vi "Read AI Channels.vi"(8 "error in (no error)":errorcluster, 11 "Task in":refnum<k21>) -> (0 "error out":errorcluster, 2 "1-Sample Average Waveforms":waveform(dbl)[](array[waveform]), 3 "Task out":refnum<k21>)   [LabVIEW 2021, in "Load Frame.lvlib"]
uses:
  Load Frame.lvlib
  <vilib>/DAQmx/miscellaneous.llb/DAQmx Fill In Error Info.vi
  <vilib>/DAQmx/read.llb/DAQmx Read (Analog 1D Wfm NChan NSamp).vi
  Acquisition/Acquisition.lvlib
  <vilib>/DAQmx/read.llb/DAQmx Read (Analog 1D Wfm NChan 1Samp).vi
panel:
  out "Unscaled Data":waveform(dbl)[](graph)
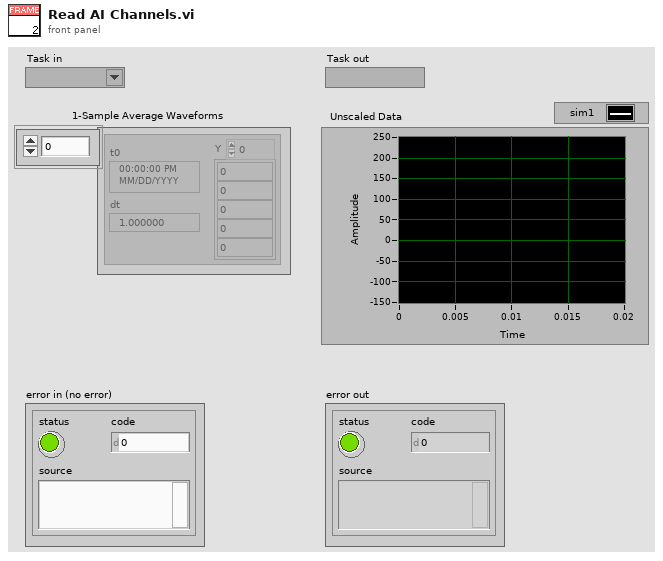
[diagram p1: front panel]
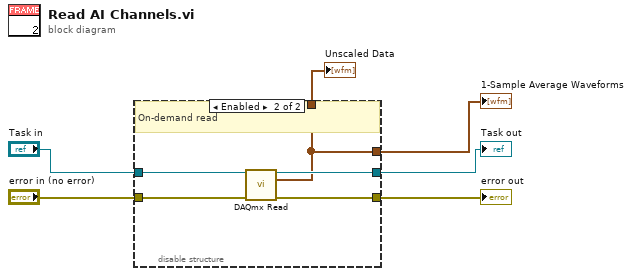
[diagram p0: block diagram]
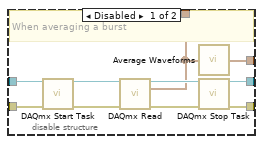
[diagram p2: hidden frame]
diagram:
  n1 = disable-structure shown="Enabled" {
    disable-tunnel: [w16 w20] -> w6
    disable-tunnel: "Task in" -> [w15 w21]
    disable-tunnel: [w14 w17] -> w4
    disable-tunnel: [w13 w19] -> w3
    disable-tunnel: "error in (no error)" -> [w9 w18]
    disable-tunnel: [w7 w17] -> w1
    frame Disabled {
      # "When averaging a burst"
      n2 = call <vilib>:"DAQmx Start Task.vi"("task/channels in"=w15, "error in"=w9) -> ("task out"=w11:refnum<k21>, "error out"=w10:errorcluster)  [unwired: 12 in]
      n3 = call-poly <vilib>:"DAQmx Read.vi"("task/channels in"=w11, "error in"=w10) -> ("task out"=w8:refnum<k21>, "data"=w7:waveform(dbl)[], "error out"=w12:errorcluster)  [unwired: 11 in]
      n4 = call "Average Waveforms.vi"("N-Sample Waveforms"=w7) -> ("1-Sample Average Waveforms"=w14:waveform(dbl)[])
      n5 = call <vilib>:"DAQmx Stop Task.vi"("task/channels in"=w8, "error in"=w12) -> ("task out"=w16:refnum<k21>, "error out"=w13:errorcluster)  [unwired: 12 in]
    }
    frame Enabled {
      # "On-demand read"
      n6 = call-poly <vilib>:"DAQmx Read.vi"("task/channels in"=w21, "error in"=w18) -> ("task out"=w20:refnum<k21>, "data"=w17:waveform(dbl)[], "error out"=w19:errorcluster)  [unwired: 11 in]
    }
  }
  "Task out" <- w6
  "1-Sample Average Waveforms" <- w4
  "error out" <- w3
  "Unscaled Data" <- w1
